vi "UDP_send_v003.vi"() -> ()   [LabVIEW 2019]
panel:
  in  "Numeric":dbl
  in  "Address List":string[][](array[string])=[["localhost", "Me"], ["192.168.1.100", "1"], ["192.168.1.103", "2"], ["192.168.1.107", "3"], ["10.60.196.72", "Fra"], ["10.60.199.221", "Albi"], ["10.60.196.113", "Greta"]]
  in  "Data to send":enum16{"String", "Numeric"}(ring)
  in  "Slide":dbl(slide) scale=0.0..10.0
  in  "Message":string
  in  "stop":bool
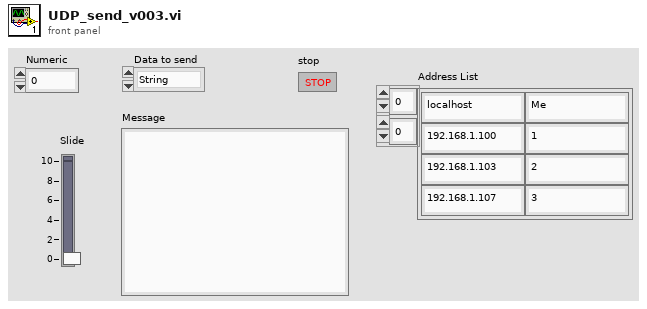
[diagram p1: front panel]
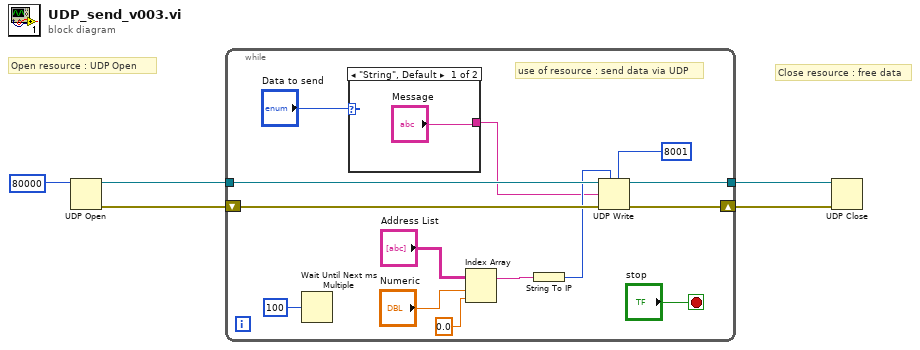
[diagram p0: block diagram]
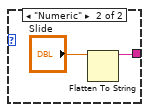
[diagram p2: hidden frame]
diagram:
  # "Close resource : free data"
  # "Open resource : UDP Open"
  n1 = UDP Open(11:80000) -> (port=w3:refnum<k16>, 0:w5:errorcluster)  [unwired: 4 in, 1 out]
  n2 = while {
    tunnel: w3 -> [w15]
    tunnel: [w14] -> w2
    shift-right: [w16] -> w4
    shift-left: w5 -> [w17]
    stop <- "stop" stop-if-true
    # "use of resource : send data via UDP"
    n3 = Wait Until Next ms Multiple(millisecond multiple=100) -> ()  [unwired: 1 out]
    n4 = case shown="\"String\", Default" "Data to send" {
      tunnel: ["Message" w21] -> w10
      frame "String", Default {
      }
      frame "Numeric" {
        n5 = Flatten To String(anything="Slide") -> (data string=w21:string)  [unwired: 3 in, 2 out]
      }
    }
    n6 = Index Array(array="Address List", index (row)="Numeric", index (col)=0.0) -> (element=w7:string)
    n7 = String To IP(1:w7) -> (0:w13:u32)
    n8 = UDP Write(address=w13, port or service name=8001, connection ID=w15, data in=w10, 8:w17) -> (error out=w16:errorcluster, 3:w14:refnum<k16>)  [unwired: 1 in]
  }
  n9 = UDP Close(connection ID=w2, 8:w4) -> ()  [unwired: 2 out]
